vi "Handwriting_DataSet.vi"() -> ()   [LabVIEW 2018]
uses:
  <vilib>/Utility/miscctls.llb/LVPositionTypeDef.ctl
  <vilib>/Utility/inputDevices.llb/mouseAcquire.vi
  <vilib>/Utility/inputDevices.llb/closeMouse.vi
panel:
  out "Break":u16
  out "Vecs":dbl[](array[numeric])
  in  "Vec_steps":u16=9
  in  "Angel File Path":path=path "C:/Users/eehys/Desktop/Angel.txt"
  in  "Vector File Path":path=path "C:/Users/eehys/Desktop/Vector.txt"
  out "Vector Seq":cluster{"Vec_Times":u16[], "Vec_CHs":u16[]}(graph)
  out "Angel Seq":cluster{"Ang_Times":u16[], "Ang_CHs":u16[]}(graph)
  out "Angel RF":cluster{"Angel":u16[], "Ang_Cnt":u16[]}(graph)
  in  "Ang_steps":u16=9
  out "Ang_CHs":u16[](array[numeric])
  out "Ang_Cnt":u16[](array[numeric])
  out "Angs":dbl[](array[numeric])
  out "Ang_Times":u16[](array[numeric])
  out "Angel":u16[](array[numeric])=[0, 1, 2, 3, 4, 5, 6, 7]
  out "Vec_Cnt":u8[](array[numeric])
  out "SmplingY":i32[](array[numeric])
  out "SmplingX":i32[](array[numeric])
  out "Y":i16[](array[numeric])
  out "X":i16[](array[numeric])
  out "Times":u32[](array[numeric])
  out "Vec_CHs":u16[](array[numeric])
  out "Vec_Times":u16[](array[numeric])
  out "Sap Count":u16
  in  "Sampling Mult":u16=5
  in  "Time step":u16=2
  out "Sets":u16
  out "Save":bool
  out "Label":u8
  in  "Save_length":u8=15
  in  "Save":bool
  out "Vector":u16[](array[numeric])=[0, 1, 2, 3, 4, 5, 6, 7]
  out "Vector RF":cluster{"Vector":u16[], "Count":u8[]}(graph)
  out "Wr_time(ms)":i16
  out "Panel":cluster{dbl[], dbl[]}[](graph)
  in  "Clear":bool
  in  "stop":bool
  # "π"
  # "Notive：\n5 * 10 for Mouse\n2 * 5 for Wacom"
  # "-π"
  # "π"
  # "-π"
  # "Time (ms)"
  # "π"
  # "-π"
  # "-π"
  # "π"
  # "Time (ms)"
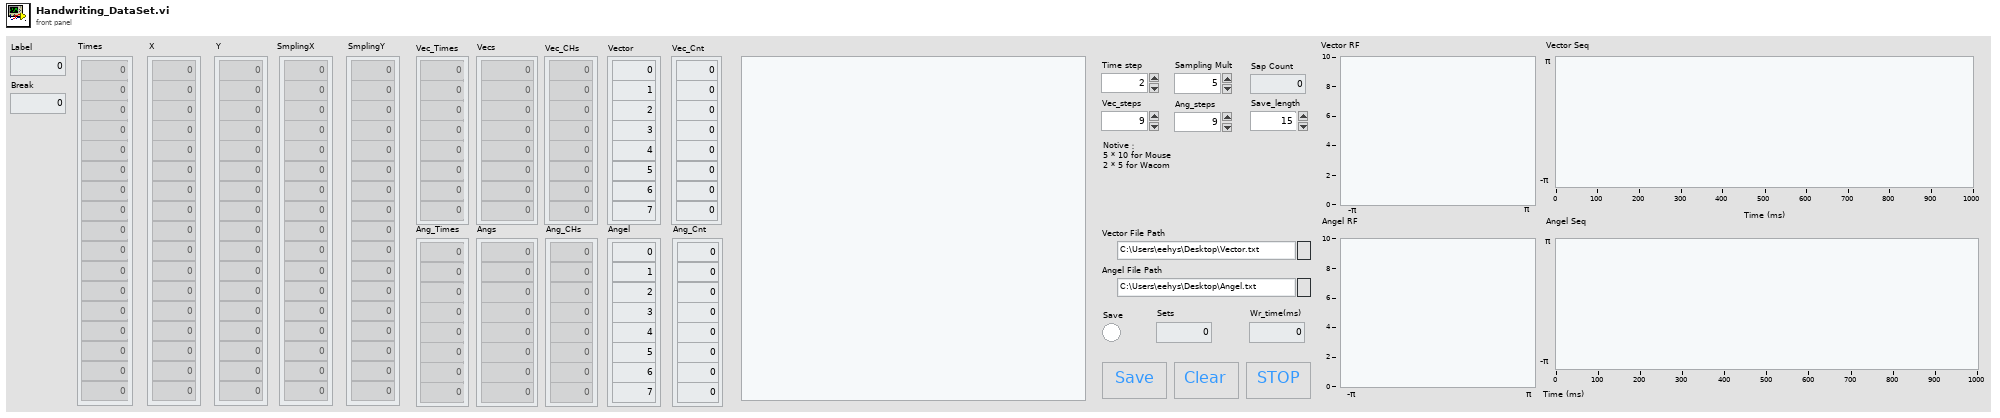
[diagram p1: front panel]
types:
  T1 = enum16{"open", "replace", "create", "open or create", "replace or create", "replace or create with confirmation"}
  T2 = typedef "LVPositionTypeDef.ctl" = cluster{"Left":i32, "Top":i32}
  T3 = cluster{"button 1":bool, "button 2":bool, "button 3":bool, "button 4":bool}
  T4 = typedef "LVPoint32TypeDef.ctl" = cluster{"Horizontal":i32, "Vertical":i32}
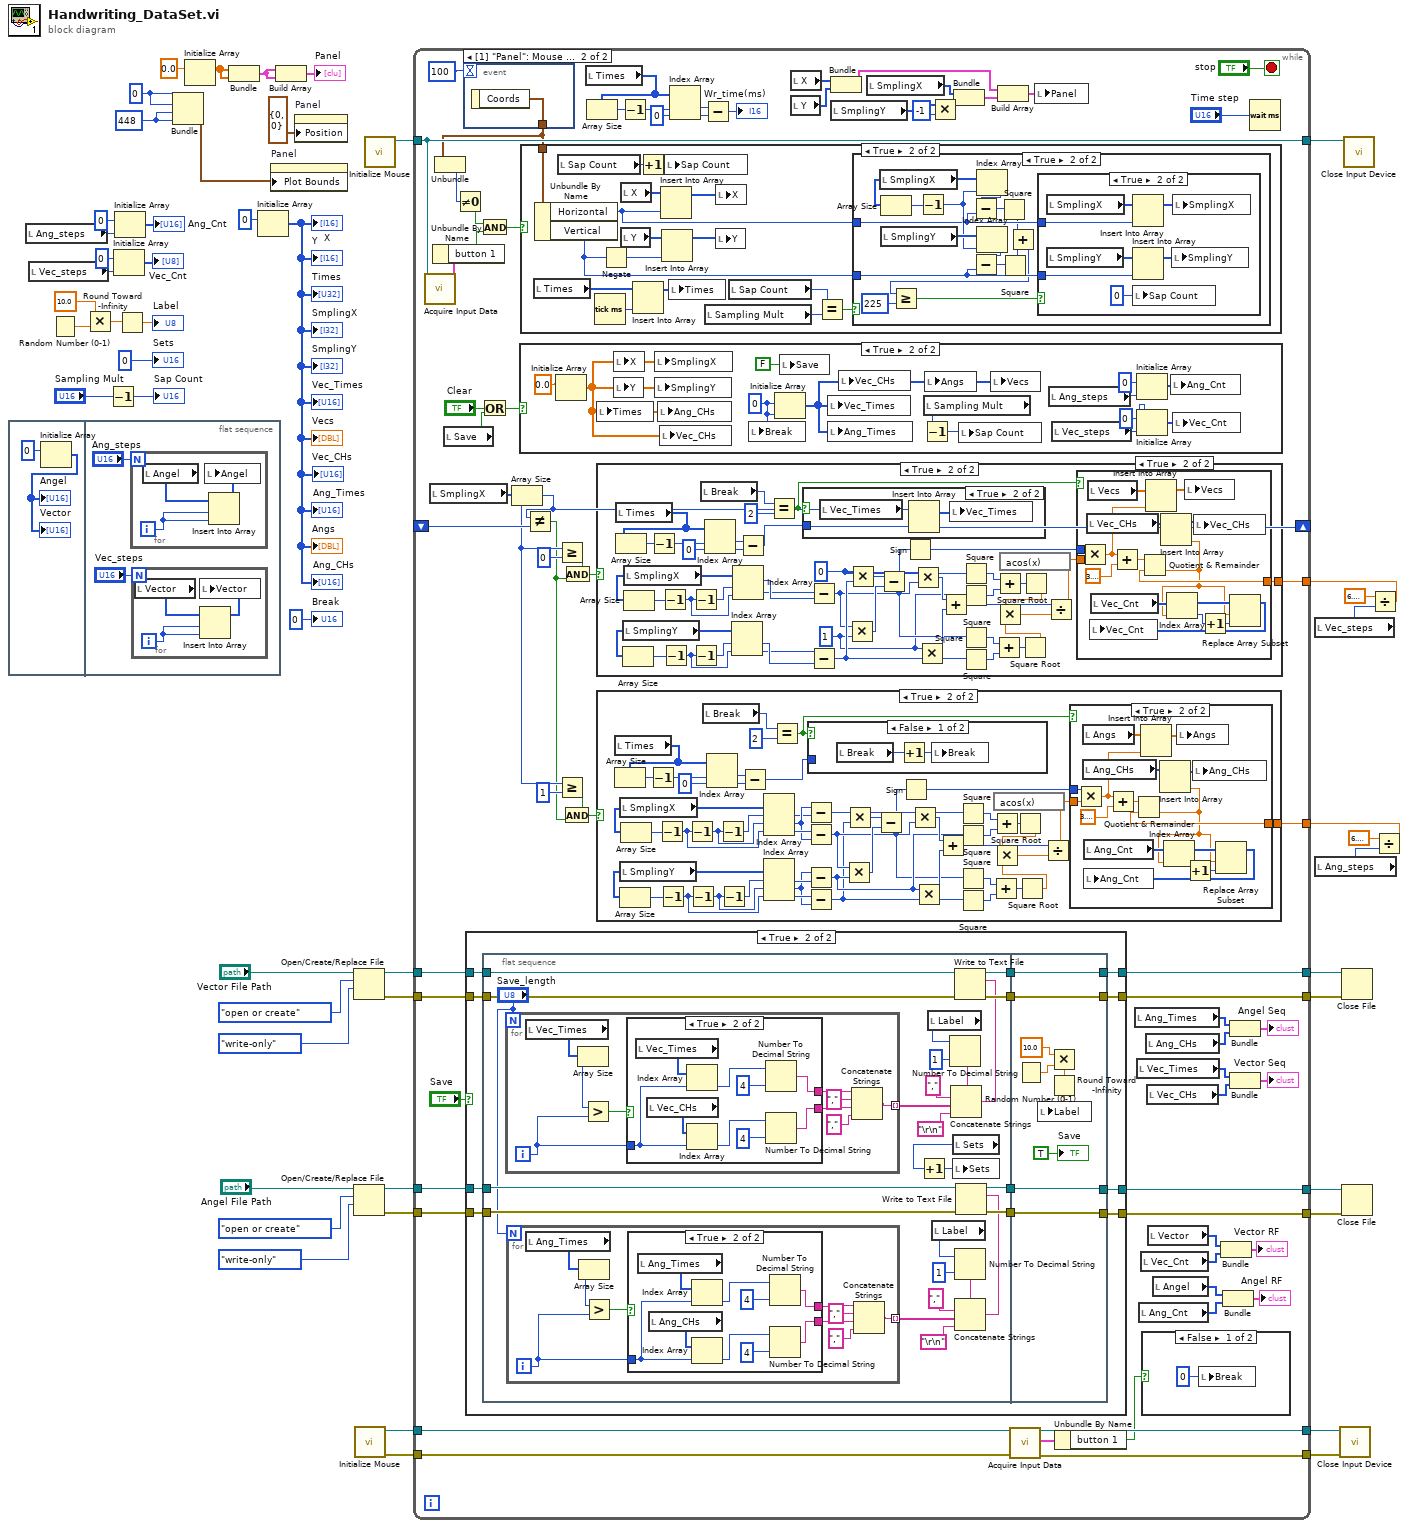
[diagram p0: block diagram]
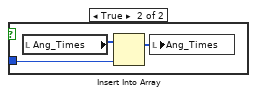
[diagram p7: hidden frame]
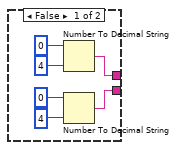
[diagram p10: hidden frame]
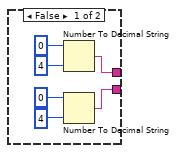
[diagram p11: hidden frame]
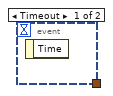
[diagram p12: hidden frame]
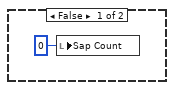
[diagram p16: hidden frame]
diagram:
  w13 = 448
  w43 = 0
  n1 = flat-sequence {
    frame #0 {
      n2 = Initialize Array(i8 0 ("element")) -> (→"Angel" →"Vector":i8[])  [unwired: 1 in]
    }
    frame #1 {
      n3 = for {
        N: "Ang_steps" -> [_]
        i -> [w58]
        n4 = local read "Angel"() -> (w59:u16[])
        n5 = Insert Into Array(array=w59, index=w58, new element=w58) -> (w60:u16[])
        n6 = local write "Angel"(w60) -> ()
      }
      n7 = for {
        N: "Vec_steps" -> [_]
        i -> [w55]
        n8 = local read "Vector"() -> (w57:u16[])
        n9 = Insert Into Array(array=w57, index=w55, new element=w55) -> (w56:u16[])
        n10 = local write "Vector"(w56) -> ()
      }
    }
  }
  n11 = local read "Ang_steps"() -> (w27:u16)
  n12 = local read "Vec_steps"() -> (w8:u16)
  n13 = Random Number (0-1)() -> (number: 0 to 1=w36:dbl)
  n14 = Multiply(x=10.0, y=w36) -> (x*y=w34:dbl)
  n15 = Decrement(x="Sampling Mult") -> (x-1=→"Sap Count":u16)
  n16 = Initialize Array(i8 0 ("element"), w8) -> (→"Vec_Cnt":i8[])
  n17 = Initialize Array(i8 0 ("element"), w27) -> (→"Ang_Cnt":i8[])
  n18 = Round Toward -Infinity(1:w34) -> (0:→"Label":dbl)
  n19 = Bundle(w43, w43, w13, w13) -> (w44:cluster{i32, i32, i32, i32})  [unwired: 1 in]
  n20 = Initialize Array(0.0 ("element")) -> (w47:dbl[])  [unwired: 1 in]
  n21 = Bundle(w47, w47) -> (w15:cluster{dbl[], dbl[]})  [unwired: 1 in]
  n22 = Initialize Array(i16 0 ("element")) -> (→"Vec_Times" →"Vec_CHs" →"Times" →"X" →"Y" →"SmplingX" →"SmplingY" →"Ang_Times" →"Angs" →"Ang_CHs" →"Vecs":i16[])  [unwired: 1 in]
  n23 = property on="Panel" class="XYGraph (strict)"("Plot Bounds"=w44) -> ()  [unwired: 2 in, 2 out]
  n24 = Build Array(w15, w15) -> (→"Panel":cluster{dbl[], dbl[]}[])
  n25 = property on="Panel" class="XYGraph (strict)"("Position"=T2 {"Left"=0, "Top"=0}) -> ()  [unwired: 2 in, 2 out]
  n26 = Open/Create/Replace File(file path (use dialog)="Vector File Path", operation (0:open)=T1."open or create", access (0:read/write)=enum16{"read/write", "read-only", "write-only"}."write-only") -> (refnum out=w40:refnum<file>, error out=w39:errorcluster)  [unwired: 3 in, 1 out]
  n27 = Open/Create/Replace File(file path (use dialog)="Angel File Path", operation (0:open)=T1."open or create", access (0:read/write)=enum16{"read/write", "read-only", "write-only"}."write-only") -> (refnum out=w19:refnum<file>, error out=w18:errorcluster)  [unwired: 3 in, 1 out]
  n28 = call <vilib>:"Initialize Mouse.vi"() -> ("error out"=w3:errorcluster, "device ID"=w5:refnum<k1>)  [unwired: 10 in]
  n29 = call <vilib>:"Initialize Mouse.vi"() -> ("device ID"=w50:refnum<k1>)  [unwired: 10 in, 1 out]
  n30 = local read "Vec_steps"() -> (w11:u16)
  n31 = local read "Ang_steps"() -> (w25:u16)
  n32 = Divide(x=6.283185307179586, y=w11) -> (x/y=w6:dbl)
  n33 = Divide(x=6.283185307179586, y=w25) -> (x/y=w24:dbl)
  n34 = while {
    tunnel: w50 -> [w127]
    tunnel: [w127] -> w49
    tunnel: w40 -> [w114]
    tunnel: w39 -> [w113]
    tunnel: [w112] -> w38
    tunnel: [w111] -> w37
    shift-right: [w77] -> _
    shift-left: _ -> [w104]
    tunnel: w24 -> [w98]
    tunnel: w19 -> [w91]
    tunnel: w18 -> [w90]
    tunnel: [w89] -> w17
    tunnel: [w88] -> w16
    tunnel: w6 -> [w67]
    tunnel: w5 -> [w66]
    tunnel: [w65] -> w4
    tunnel: w3 -> [w64]
    tunnel: [w63] -> w2
    stop <- "stop" stop-if-true
    n35 = call-poly <vilib>:"Acquire Input Data.vi"("device ID"=w127) -> ("button info"=w126:T3)  [unwired: 15 in, 3 out]
    n36 = local read "SmplingX"() -> (w105:i32[])
    n37 = Unbundle By Name(w126) -> ("button 1"=w116:bool)
    n38 = local read "Save"() -> (w107:bool)
    n39 = event shown="[1] \"Panel\": Mouse Move" {
      selector: _ -> [_ _]
      dyn-events: _ -> [_ _]
      timeout: 100 -> [_ _]
      tunnel: [_ w360] -> w119
      event Timeout {
        n40 = event-data() -> ()  [unwired: 1 in, 1 out]
      }
      event "Panel": Mouse Move {
        n41 = event-data() -> ("Coords"=w360:T4)  [unwired: 1 in]
      }
    }
    n42 = Unbundle(w119) -> ("Vertical"=w118:i32)  [unwired: 1 out]
    n43 = Not Equal To 0?(x=w118) -> (x != 0?=w117:bool)
    n44 = case shown="True" "Save" {
      tunnel: w114 -> [w265 w277]
      tunnel: w113 -> [w264 w276]
      tunnel: [w265 w275] -> w112
      tunnel: [w264 w274] -> w111
      tunnel: w91 -> [w263 w271]
      tunnel: w90 -> [w262 w270]
      tunnel: [w263 w268] -> w89
      tunnel: [w262 w266] -> w88
      frame False {
      }
      frame True {
        n45 = flat-sequence {
          tunnel: w277 -> [w302]
          tunnel: w276 -> [w301]
          tunnel: [w300] -> w273
          tunnel: [w299] -> w272
          tunnel: w271 -> [w283]
          tunnel: w270 -> [w282]
          tunnel: [w285] -> w269
          tunnel: [w284] -> w267
          tunnel: [w358] -> w274
          tunnel: [w359] -> w275
          tunnel: w273 -> [w359]
          tunnel: w272 -> [w358]
          tunnel: w269 -> [w352]
          tunnel: [w352] -> w268
          tunnel: w267 -> [w351]
          tunnel: [w351] -> w266
          frame #0 {
            n46 = for {
              N: "Save_length" -> [_]
              tunnel: [w330] -> w293 mode=indexing
              i -> [w327]
              n47 = local read "Vec_Times"() -> (w335:u16[])
              n48 = Array Size(array=w335) -> (size(s)=w334:i32)
              n49 = Greater?(x=w334, y=w327) -> (0:w333:bool)
              n50 = case shown="True" w333 {
                tunnel: [w337 w348] -> w329
                tunnel: [w336 w347] -> w328
                tunnel: w327 -> [_ w342]
                frame False {
                  n51 = Number To Decimal String(number=0, width (-)=i16 4) -> (decimal integer string=w337:string)
                  n52 = Number To Decimal String(number=0, width (-)=i16 4) -> (decimal integer string=w336:string)
                }
                frame True {
                  n53 = local read "Vec_Times"() -> (w344:u16[])
                  n54 = local read "Vec_CHs"() -> (w343:u16[])
                  n55 = Index Array(array=w344, index=w342) -> (element=w345:u16)
                  n56 = Index Array(array=w343, index=w342) -> (element=w346:u16)
                  n57 = Number To Decimal String(number=w345, width (-)=i16 4) -> (decimal integer string=w348:string)
                  n58 = Number To Decimal String(number=w346, width (-)=i16 4) -> (decimal integer string=w347:string)
                }
              }
              n59 = Concatenate Strings(w329, "," ("string"), w328, "," ("string")) -> (w330:string)
            }
            n60 = for {
              N: "Save_length" -> [_]
              tunnel: [w303] -> w280 mode=indexing
              i -> [w308]
              n61 = local read "Ang_Times"() -> (w311:u16[])
              n62 = Array Size(array=w311) -> (size(s)=w310:i32)
              n63 = Greater?(x=w310, y=w308) -> (0:w309:bool)
              n64 = case shown="True" w309 {
                tunnel: w308 -> [_ w324]
                tunnel: [w313 w319] -> w305
                tunnel: [w312 w318] -> w304
                frame False {
                  n65 = Number To Decimal String(number=0, width (-)=i16 4) -> (decimal integer string=w313:string)
                  n66 = Number To Decimal String(number=0, width (-)=i16 4) -> (decimal integer string=w312:string)
                }
                frame True {
                  n67 = local read "Ang_Times"() -> (w326:u16[])
                  n68 = local read "Ang_CHs"() -> (w325:u16[])
                  n69 = Index Array(array=w326, index=w324) -> (element=w320:u16)
                  n70 = Index Array(array=w325, index=w324) -> (element=w321:u16)
                  n71 = Number To Decimal String(number=w320, width (-)=i16 4) -> (decimal integer string=w319:string)
                  n72 = Number To Decimal String(number=w321, width (-)=i16 4) -> (decimal integer string=w318:string)
                }
              }
              n73 = Concatenate Strings(w305, "," ("string"), w304, "," ("string")) -> (w303:string)
            }
            n74 = local read "Label"() -> (w292:u8)
            n75 = local read "Label"() -> (w281:u8)
            n76 = Number To Decimal String(number=w292, width (-)=i16 1) -> (decimal integer string=w295:string)
            n77 = Concatenate Strings(w295, "," ("string"), w293, "\r\n") -> (w294:string)
            n78 = local read "Sets"() -> (w290:u16)
            n79 = Increment(x=w290) -> (x+1=w291:u16)
            n80 = local write "Sets"(w291) -> ()
            n81 = Write to Text File(file (use dialog)=w302, text=w294, error in=w301) -> (refnum out=w300:refnum<file>, error out=w299:errorcluster)  [unwired: 1 in, 1 out]
            n82 = Number To Decimal String(number=w281, width (-)=i16 1) -> (decimal integer string=w286:string)
            n83 = Concatenate Strings(w286, "," ("string"), w280, "\r\n") -> (w279:string)
            n84 = Write to Text File(file (use dialog)=w283, text=w279, error in=w282) -> (refnum out=w285:refnum<file>, error out=w284:errorcluster)  [unwired: 1 in, 1 out]
          }
          frame #1 {
            n85 = Random Number (0-1)() -> (number: 0 to 1=w357:dbl)
            n86 = Multiply(x=10.0, y=w357) -> (x*y=w355:dbl)
            n87 = Round Toward -Infinity(1:w355) -> (0:w354:dbl)
            n88 = local write "Label"(w354) -> ()
            "Save" <- TRUE ("Save")
          }
        }
      }
    }
    n89 = And(x=w117, y=w116) -> (x .and. y?=w115:bool)
    n90 = Or(x="Clear", y=w107) -> (x .or. y?=w110:bool)
    n91 = Array Size(array=w105) -> (size(s)=w77:i32)
    n92 = case shown="True" w110 {
      frame False {
      }
      frame True {
        w361 = u8 0 ("element")
        n93 = Initialize Array(0.0 ("element")) -> (w368:dbl[])  [unwired: 1 in]
        n94 = local write "Times"(w368) -> ()
        n95 = local write "X"(w368) -> ()
        n96 = local write "Y"(w368) -> ()
        n97 = local write "SmplingX"(w368) -> ()
        n98 = local write "SmplingY"(w368) -> ()
        n99 = local write "Ang_CHs"(w368) -> ()
        n100 = local write "Vec_CHs"(w368) -> ()
        n101 = local write "Break"(w361) -> ()
        n102 = Initialize Array(w361, w361) -> (w369:u8[])
        n103 = local write "Save"(FALSE ("SaveSta")) -> ()
        n104 = local write "Vec_Times"(w369) -> ()
        n105 = local write "Ang_Times"(w369) -> ()
        n106 = local write "Vec_CHs"(w369) -> ()
        n107 = local read "Sampling Mult"() -> (w370:u16)
        n108 = Decrement(x=w370) -> (x-1=w371:u16)
        n109 = local write "Angs"(w369) -> ()
        n110 = local write "Sap Count"(w371) -> ()
        n111 = local write "Vecs"(w369) -> ()
        n112 = local read "Ang_steps"() -> (w367:u16)
        n113 = local read "Vec_steps"() -> (w365:u16)
        n114 = Initialize Array(i8 0 ("element"), w367) -> (w366:i8[])
        n115 = Initialize Array(u8 0 ("element"), w365) -> (w364:u8[])
        n116 = local write "Ang_Cnt"(w366) -> ()
        n117 = local write "Vec_Cnt"(w364) -> ()
      }
    }
    n118 = case shown="True" w115 {
      tunnel: w119 -> [_ w385]
      frame False {
      }
      frame True {
        n119 = local read "Times"() -> (w384:u32[])
        n120 = Unbundle By Name(w385) -> ("Horizontal"=w378:i32, "Vertical"=w376:i32)
        n121 = local read "Sap Count"() -> (w381:u16)
        n122 = Tick Count (ms)() -> (millisecond timer value=w382:u32)
        n123 = Negate(x=w376) -> (-x=w377:i32)
        n124 = local read "X"() -> (w389:i16[])
        n125 = local read "Y"() -> (w388:i16[])
        n126 = Insert Into Array(array=w384, new element=w382) -> (w383:u32[])  [unwired: 1 in]
        n127 = Increment(x=w381) -> (x+1=w380:u16)
        n128 = Insert Into Array(array=w389, new element=w378) -> (w387:i16[])  [unwired: 1 in]
        n129 = Insert Into Array(array=w388, new element=w377) -> (w386:i16[])  [unwired: 1 in]
        n130 = local write "Sap Count"(w380) -> ()
        n131 = local write "Times"(w383) -> ()
        n132 = local read "Sampling Mult"() -> (w375:u16)
        n133 = local write "X"(w387) -> ()
        n134 = local write "Y"(w386) -> ()
        n135 = local read "Sap Count"() -> (w379:u16)
        n136 = Equal?(x=w379, y=w375) -> (x = y?=w374:bool)
        n137 = case shown="True" w374 {
          tunnel: w378 -> [_ w399]
          tunnel: w376 -> [_ w397]
          frame False {
          }
          frame True {
            n138 = local read "SmplingX"() -> (w403:i32[])
            n139 = Array Size(array=w403) -> (size(s)=w402:i32)
            n140 = local read "SmplingY"() -> (w404:i32[])
            n141 = Decrement(x=w402) -> (x-1=w401:i32)
            n142 = Index Array(array=w403, index=w401) -> (element=w400:i32)
            n143 = Subtract(x=w400, y=w399) -> (x-y=w396:i32)
            n144 = Index Array(array=w404, index=w401) -> (element=w398:i32)
            n145 = Subtract(x=w398, y=w397) -> (x-y=w395:i32)
            n146 = Square(x=w396) -> (x^2=w394:i32)
            n147 = Square(x=w395) -> (x^2=w393:i32)
            n148 = Add(x=w394, y=w393) -> (x+y=w392:i32)
            n149 = Greater Or Equal?(x=w392, y=225) -> (x >= y?=w390:bool)
            n150 = case shown="True" w390 {
              tunnel: w399 -> [_ w408]
              tunnel: w397 -> [_ w406]
              frame False {
                n151 = local write "Sap Count"(u16 0 ("Sap Count")) -> ()
              }
              frame True {
                n152 = local read "SmplingX"() -> (w412:i32[])
                n153 = local read "SmplingY"() -> (w410:i32[])
                n154 = Insert Into Array(array=w412, new element=w408) -> (w411:i32[])  [unwired: 1 in]
                n155 = Insert Into Array(array=w410, new element=w406) -> (w409:i32[])  [unwired: 1 in]
                n156 = local write "Sap Count"(u16 0 ("Sp Mt Ct")) -> ()
                n157 = local write "SmplingY"(w409) -> ()
                n158 = local write "SmplingX"(w411) -> ()
              }
            }
          }
        }
      }
    }
    n159 = Not Equal?(x=w77, y=w104) -> (x != y?=w75:bool)
    n160 = Greater Or Equal?(x=w77, y=0) -> (x >= y?=w74:bool)
    n161 = Greater Or Equal?(x=w77, y=1) -> (x >= y?=w99:bool)
    n162 = And(x=w99, y=w75) -> (x .and. y?=w100:bool)
    n163 = And(x=w74, y=w75) -> (x .and. y?=w76:bool)
    n164 = local read "Times"() -> (w124:u32[])
    n165 = Array Size(array=w124) -> (size(s)=w102:i32)
    n166 = case shown="True" w76 {
      tunnel: w67 -> [_ w138]
      frame False {
      }
      frame True {
        w140 = 0
        w139 = 1 ("y")
        n167 = local read "Times"() -> (w169:u32[])
        n168 = Array Size(array=w169) -> (size(s)=w171:i32)
        n169 = local read "SmplingY"() -> (w156:i32[])
        n170 = Array Size(array=w156) -> (size(s)=w157:i32)
        n171 = local read "SmplingX"() -> (w158:i32[])
        n172 = Array Size(array=w158) -> (size(s)=w159:i32)
        n173 = Decrement(x=w171) -> (x-1=w170:i32)
        n174 = Decrement(x=w159) -> (x-1=w135:i32)
        n175 = Decrement(x=w157) -> (x-1=w133:i32)
        n176 = Decrement(x=w135) -> (x-1=w136:i32)
        n177 = Decrement(x=w133) -> (x-1=w134:i32)
        n178 = local read "Break"() -> (w132:u16)
        n179 = Index Array(array=w169, index #1=w170, index #2=0 ("index")) -> (element #1=w173:u32, element #2=w172:u32)
        n180 = Index Array(array=w156, index #1=w134, index #2=w133) -> (element #1=w153:i32, element #2=w152:i32)
        n181 = Index Array(array=w158, index #1=w136, index #2=w135) -> (element #1=w155:i32, element #2=w154:i32)
        n182 = Subtract(x=w173, y=w172) -> (x-y=w168:u32)
        n183 = Equal?(x=w132, y=u16 2) -> (x = y?=w130:bool)
        n184 = case shown="True" w130 {
          tunnel: w168 -> [_ w176]
          frame False {
          }
          frame True {
            n185 = local read "Vec_Times"() -> (w177:u16[])
            n186 = Insert Into Array(array=w177, new element=w176) -> (w175:u16[])  [unwired: 1 in]
            n187 = local write "Vec_Times"(w175) -> ()
          }
        }
        n188 = Subtract(x=w154, y=w155) -> (x-y=w150:i32)
        n189 = Subtract(x=w152, y=w153) -> (x-y=w161:i32)
        n190 = Multiply(x=w150, y=w139) -> (x*y=w167:i32)
        n191 = Multiply(x=w140, y=w161) -> (x*y=w166:i32)
        n192 = Subtract(x=w166, y=w167) -> (x-y=w151:i32)
        n193 = Sign(1:w151) -> (0:w141:i32)
        n194 = Multiply(x=w140, y=w150) -> (x*y=w149:i32)
        n195 = Multiply(x=w139, y=w161) -> (x*y=w162:i32)
        n196 = Add(x=w149, y=w162) -> (x+y=w145:i32)
        n197 = Square(x=w140) -> (x^2=w148:i32)
        n198 = Square(x=w139) -> (x^2=w147:i32)
        n199 = Square(x=w150) -> (x^2=w160:i32)
        n200 = Square(x=w161) -> (x^2=w165:i32)
        n201 = Add(x=w160, y=w165) -> (x+y=w164:i32)
        n202 = Add(x=w148, y=w147) -> (x+y=w137:i32)
        n203 = Square Root(x=w164) -> (sqrt(x)=w163:dbl)
        n204 = Square Root(x=w137) -> (sqrt(x)=w146:dbl)
        n205 = Multiply(x=w146, y=w163) -> (x*y=w144:dbl)
        n206 = Divide(x=w145, y=w144) -> (x/y=w143:dbl)
        n207 = expression code="acos(x)"(w143) -> (w142:dbl)
        n208 = case shown="True" w130 {
          tunnel: w142 -> [_ w187]
          tunnel: w141 -> [_ w186]
          tunnel: w138 -> [_ w179]
          frame False {
          }
          frame True {
            n209 = Multiply(x=w186, y=w187) -> (x*y=w184:dbl)
            n210 = local read "Vec_CHs"() -> (w189:u16[])
            n211 = local read "Vecs"() -> (w190:dbl[])
            n212 = local read "Vec_Cnt"() -> (w182:u8[])
            n213 = Add(x=w184, y=3.141592653589793) -> (x+y=w183:dbl)
            n214 = Quotient & Remainder(x=w183, y=w179) -> (floor(x/y)=w178:dbl)  [unwired: 1 out]
            n215 = Insert Into Array(array=w190, new element=w184) -> (w191:dbl[])  [unwired: 1 in]
            n216 = Insert Into Array(array=w189, new element=w178) -> (w188:u16[])  [unwired: 1 in]
            n217 = Index Array(array=w182, index=w178) -> (element=w181:u8)
            n218 = local write "Vecs"(w191) -> ()
            n219 = local write "Vec_CHs"(w188) -> ()
            n220 = Increment(x=w181) -> (x+1=w192:u8)
            n221 = Replace Array Subset(array=w182, new element=w192, index=w178) -> (w180:u8[])
            n222 = local write "Vec_Cnt"(w180) -> ()
          }
        }
      }
    }
    n223 = case shown="True" w100 {
      tunnel: w98 -> [_ w198]
      frame False {
      }
      frame True {
        n224 = local read "Times"() -> (w236:u32[])
        n225 = Array Size(array=w236) -> (size(s)=w238:i32)
        n226 = local read "SmplingX"() -> (w233:i32[])
        n227 = local read "SmplingY"() -> (w231:i32[])
        n228 = Array Size(array=w231) -> (size(s)=w232:i32)
        n229 = Array Size(array=w233) -> (size(s)=w234:i32)
        n230 = Decrement(x=w238) -> (x-1=w237:i32)
        n231 = Decrement(x=w234) -> (x-1=w227:i32)
        n232 = Decrement(x=w232) -> (x-1=w222:i32)
        n233 = Decrement(x=w227) -> (x-1=w225:i32)
        n234 = Decrement(x=w222) -> (x-1=w223:i32)
        n235 = local read "Break"() -> (w195:u16)
        n236 = Index Array(array=w236, index #1=w237, index #2=0 ("index")) -> (element #1=w240:u32, element #2=w239:u32)
        n237 = Decrement(x=w225) -> (x-1=w226:i32)
        n238 = Decrement(x=w223) -> (x-1=w224:i32)
        n239 = Subtract(x=w240, y=w239) -> (x-y=w235:u32)
        n240 = Index Array(array=w233, index #1=w226, index #2=w225, index #3=w227) -> (element #1=w219:i32, element #2=w220:i32, element #3=w221:i32)
        n241 = Index Array(array=w231, index #1=w224, index #2=w223, index #3=w222) -> (element #1=w230:i32, element #2=w228:i32, element #3=w229:i32)
        n242 = Equal?(x=w195, y=u16 2) -> (x = y?=w193:bool)
        n243 = Subtract(x=w220, y=w219) -> (x-y=w207:i32)
        n244 = Subtract(x=w221, y=w220) -> (x-y=w205:i32)
        n245 = Subtract(x=w228, y=w230) -> (x-y=w206:i32)
        n246 = Subtract(x=w229, y=w228) -> (x-y=w204:i32)
        n247 = case shown="False" w193 {
          tunnel: w235 -> [_ w244]
          frame False {
            n248 = local read "Break"() -> (w243:u16)
            n249 = Increment(x=w243) -> (x+1=w242:u16)
            n250 = local write "Break"(w242) -> ()
          }
          frame True {
            n251 = local read "Ang_Times"() -> (w246:u16[])
            n252 = Insert Into Array(array=w246, new element=w244) -> (w245:u16[])  [unwired: 1 in]
            n253 = local write "Ang_Times"(w245) -> ()
          }
        }
        n254 = Multiply(x=w205, y=w206) -> (x*y=w218:i32)
        n255 = Multiply(x=w207, y=w204) -> (x*y=w217:i32)
        n256 = Subtract(x=w217, y=w218) -> (x-y=w200:i32)
        n257 = Sign(1:w200) -> (0:w199:i32)
        n258 = Multiply(x=w207, y=w205) -> (x*y=w209:i32)
        n259 = Multiply(x=w206, y=w204) -> (x*y=w208:i32)
        n260 = Add(x=w209, y=w208) -> (x+y=w211:i32)
        n261 = Square(x=w207) -> (x^2=w215:i32)
        n262 = Square(x=w206) -> (x^2=w203:i32)
        n263 = Square(x=w205) -> (x^2=w202:i32)
        n264 = Square(x=w204) -> (x^2=w214:i32)
        n265 = Add(x=w202, y=w214) -> (x+y=w196:i32)
        n266 = Add(x=w215, y=w203) -> (x+y=w216:i32)
        n267 = Square Root(x=w216) -> (sqrt(x)=w213:dbl)
        n268 = Square Root(x=w196) -> (sqrt(x)=w212:dbl)
        n269 = Multiply(x=w213, y=w212) -> (x*y=w197:dbl)
        n270 = Divide(x=w211, y=w197) -> (x/y=w210:dbl)
        n271 = expression code="acos(x)"(w210) -> (w201:dbl)
        n272 = case shown="True" w193 {
          tunnel: w201 -> [_ w259]
          tunnel: w199 -> [_ w258]
          tunnel: w198 -> [_ w252]
          frame False {
          }
          frame True {
            n273 = Multiply(x=w258, y=w259) -> (x*y=w255:dbl)
            n274 = local read "Angs"() -> (w261:dbl[])
            n275 = local read "Ang_CHs"() -> (w256:u16[])
            n276 = local read "Ang_Cnt"() -> (w251:u16[])
            n277 = Add(x=w255, y=3.141592653589793) -> (x+y=w253:dbl)
            n278 = Quotient & Remainder(x=w253, y=w252) -> (floor(x/y)=w249:dbl)  [unwired: 1 out]
            n279 = Insert Into Array(array=w261, new element=w255) -> (w260:dbl[])  [unwired: 1 in]
            n280 = Insert Into Array(array=w256, new element=w249) -> (w257:u16[])  [unwired: 1 in]
            n281 = Index Array(array=w251, index=w249) -> (element=w247:u16)
            n282 = local write "Angs"(w260) -> ()
            n283 = Increment(x=w247) -> (x+1=w248:u16)
            n284 = local write "Ang_CHs"(w257) -> ()
            n285 = Replace Array Subset(array=w251, new element=w248, index=w249) -> (w250:u16[])
            n286 = local write "Ang_Cnt"(w250) -> ()
          }
        }
      }
    }
    n287 = Decrement(x=w102) -> (x-1=w101:i32)
    n288 = Index Array(array=w124, index #1=w101, index #2=0 ("index")) -> (element #1=w122:u32, element #2=w121:u32)
    n289 = Subtract(x=w122, y=w121) -> (x-y=→"Wr_time(ms)":u32)
    n290 = local read "X"() -> (w87:i16[])
    n291 = local read "Y"() -> (w86:i16[])
    n292 = Bundle("X"=w87, "Y"=w86) -> (w81:cluster{"X":i16[], "Y":i16[]})  [unwired: 1 in]
    n293 = local read "SmplingY"() -> (w83:i32[])
    n294 = local read "SmplingX"() -> (w85:i32[])
    n295 = Multiply(x=w83, y=-1) -> (x*y=w82:i32[])
    n296 = Bundle("SmplingX"=w85, w82) -> (w80:cluster{"SmplingX":i32[], i32[]})  [unwired: 1 in]
    n297 = Build Array(w81, w80) -> (w79:cluster{"SmplingX":i32[], "Y":i32[]}[])
    n298 = call-poly <vilib>:"Acquire Input Data.vi"("device ID"=w66, "error in (no error)"=w64) -> ("device ID"=w65:refnum<k1>, "button info"=w62:T3, "error out"=w63:errorcluster)  [unwired: 14 in, 1 out]
    n299 = local write "Panel"(w79) -> ()
    n300 = Unbundle By Name(w62) -> ("button 1"=w61:bool)
    n301 = local read "Ang_Times"() -> (w96:u16[])
    n302 = local read "Vec_Times"() -> (w94:u16[])
    n303 = local read "Ang_Cnt"() -> (w69:u16[])
    n304 = local read "Vec_Cnt"() -> (w72:u8[])
    n305 = case shown="False" w61 {
      frame False {
        n306 = local write "Break"(u16 0 ("Break")) -> ()
      }
      frame True {
      }
    }
    n307 = local read "Ang_CHs"() -> (w95:u16[])
    n308 = local read "Vec_CHs"() -> (w93:u16[])
    n309 = local read "Vector"() -> (w73:u16[])
    n310 = local read "Angel"() -> (w68:u16[])
    n311 = Bundle("Vector"=w73, "Vec_Cnt"=w72) -> (→"Vector RF":cluster{"Vector":u16[], "Vec_Cnt":u8[]})  [unwired: 1 in]
    n312 = Bundle("Angel"=w68, "Ang_Cnt"=w69) -> (→"Angel RF":cluster{"Angel":u16[], "Ang_Cnt":u16[]})  [unwired: 1 in]
    n313 = Bundle("Ang_Times"=w96, "Ang_CHs"=w95) -> (→"Angel Seq":cluster{"Ang_Times":u16[], "Ang_CHs":u16[]})  [unwired: 1 in]
    n314 = Bundle("Vec_Times"=w94, "Vec_CHs"=w93) -> (→"Vector Seq":cluster{"Vec_Times":u16[], "Vec_CHs":u16[]})  [unwired: 1 in]
    n315 = Wait (ms)(milliseconds to wait="Time step") -> ()  [unwired: 1 out]
  }
  n316 = call-poly <vilib>:"Close Input Device.vi"("error in (no error)"=w2, "device ID"=w4) -> ()  [unwired: 8 in, 1 out]
  n317 = Close File(refnum=w38, error in=w37) -> ()  [unwired: 2 out]
  n318 = Close File(refnum=w17, error in=w16) -> ()  [unwired: 2 out]
  n319 = call-poly <vilib>:"Close Input Device.vi"("device ID"=w49) -> ()  [unwired: 9 in, 1 out]
  "Sets" <- u8 0 ("Data Sets")
  "Break" <- u16 0 ("Break")
